vi "Cube_Intensity_png.vi"(3 "No of Contours":i32=20, 4 "Job Directory":path=path "/Lacie_20/paulhayden/Documents/EnFlo bits/EnFlo Tun Vel profiles/View_LDA data.tpt", 5 "Intensity Graph":dbl[][](graph)) -> ()   [LabVIEW 2011]
uses:
  Results_plotter_Global.vi
panel:
  in  "Save Automatically?":bool
  in  "Auto scale Intensity":bool=TRUE
  in  "Colour":bool=TRUE
  out "Results Filename":string
  out "Date":string
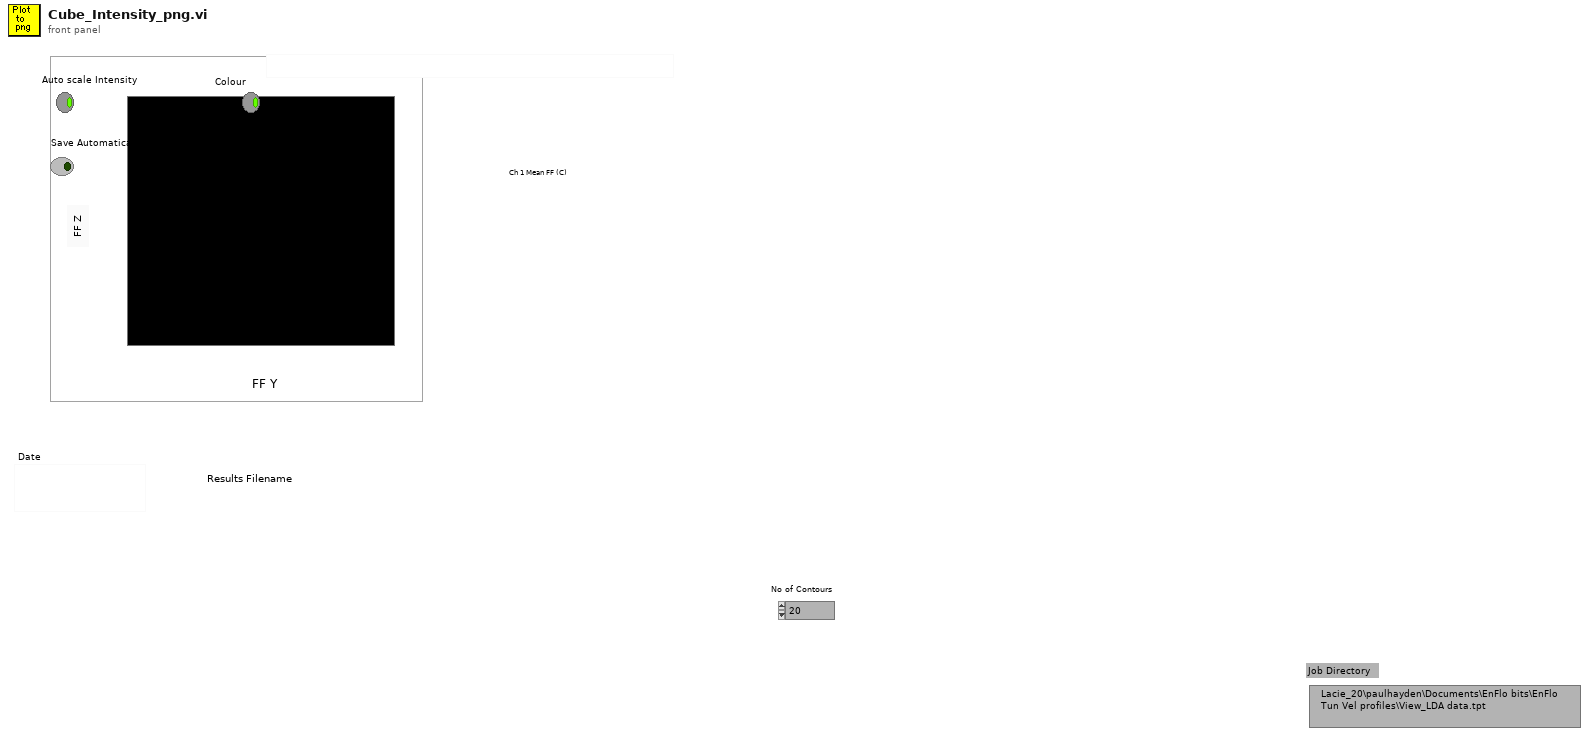
[diagram p1: front panel]
types:
  T1 = typedef "LVRectTypeDef.ctl" = cluster{"left":i16, "top":i16, "right":i16, "bottom":i16}
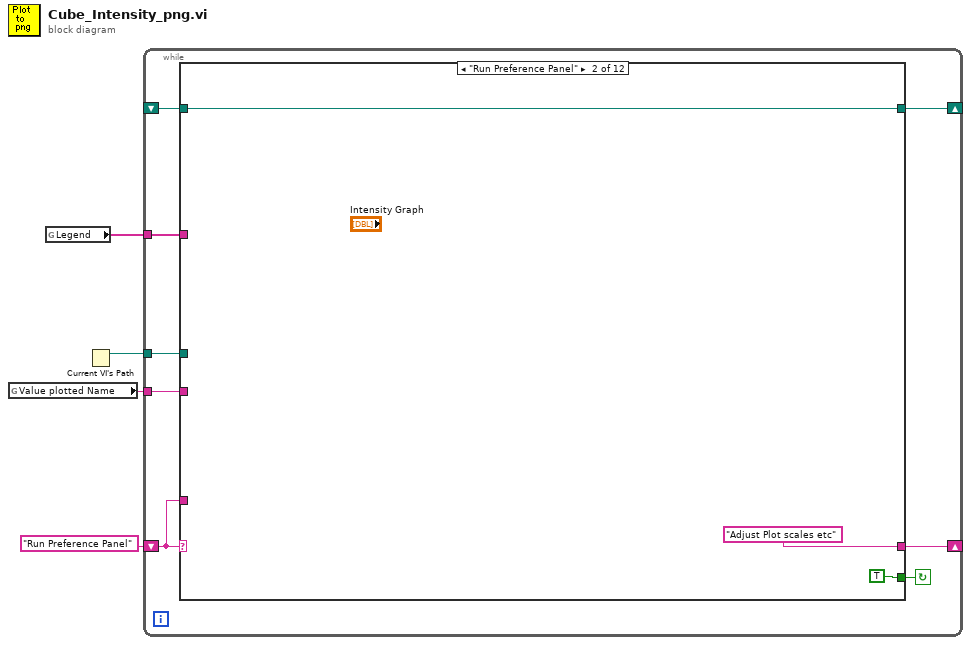
[diagram p0: block diagram]
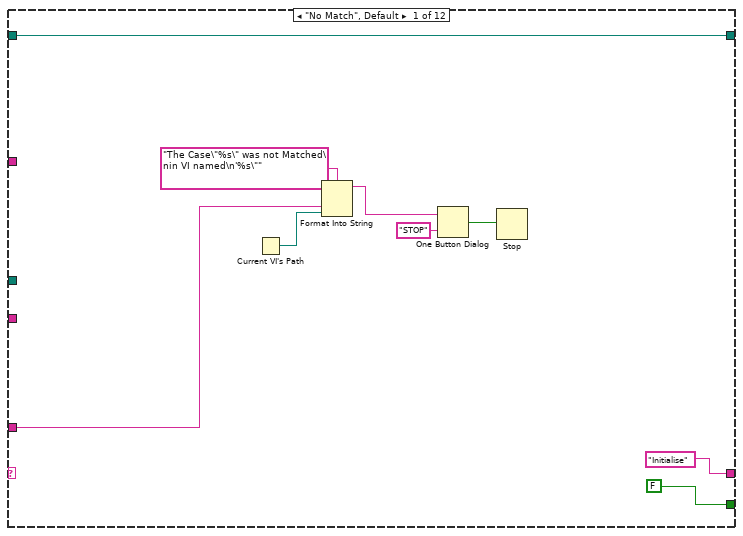
[diagram p2: hidden frame]
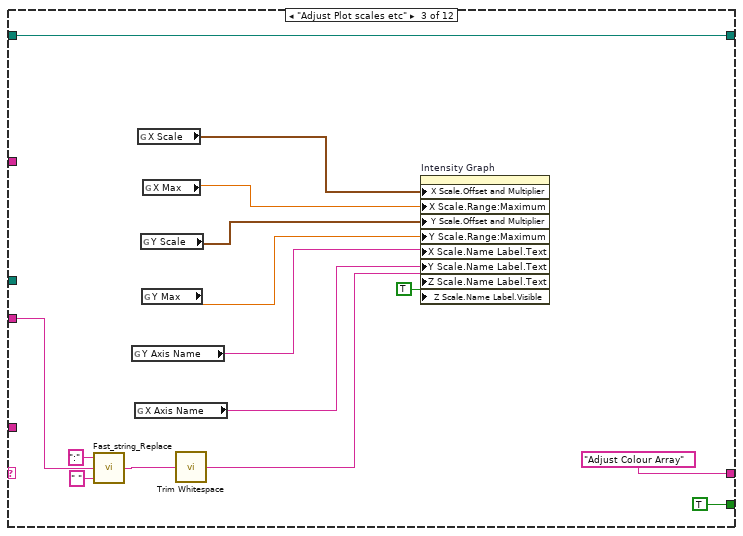
[diagram p3: hidden frame]
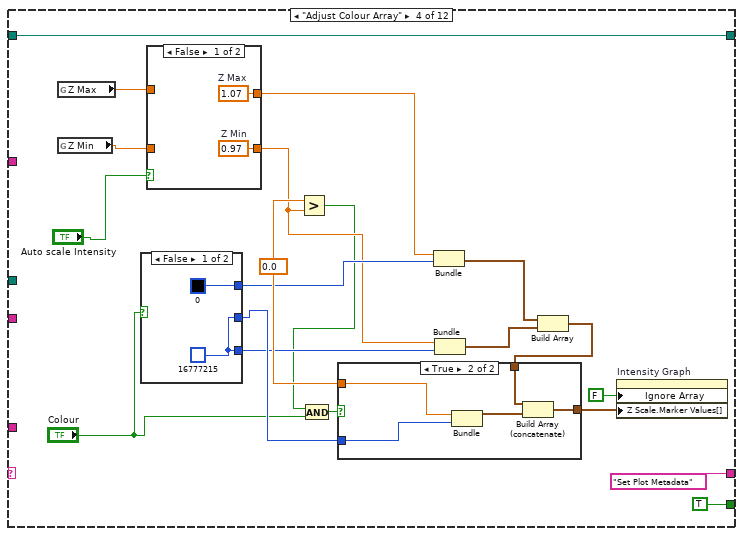
[diagram p4: hidden frame]
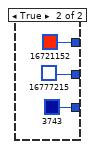
[diagram p5: hidden frame]
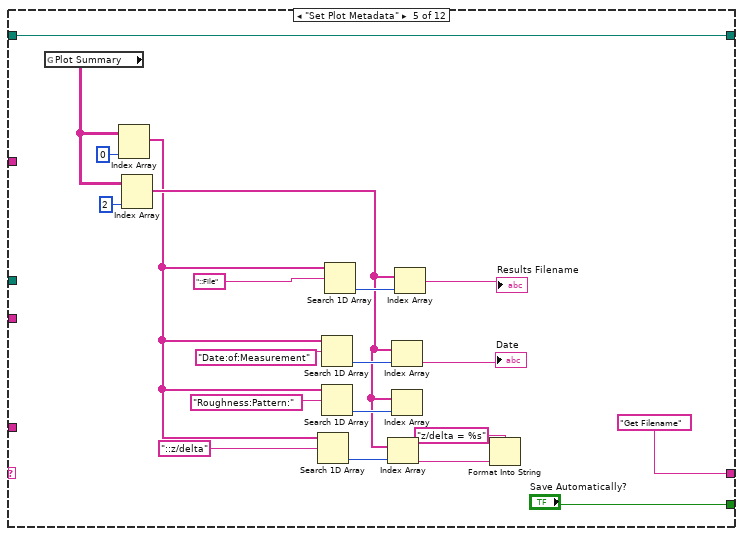
[diagram p8: hidden frame]
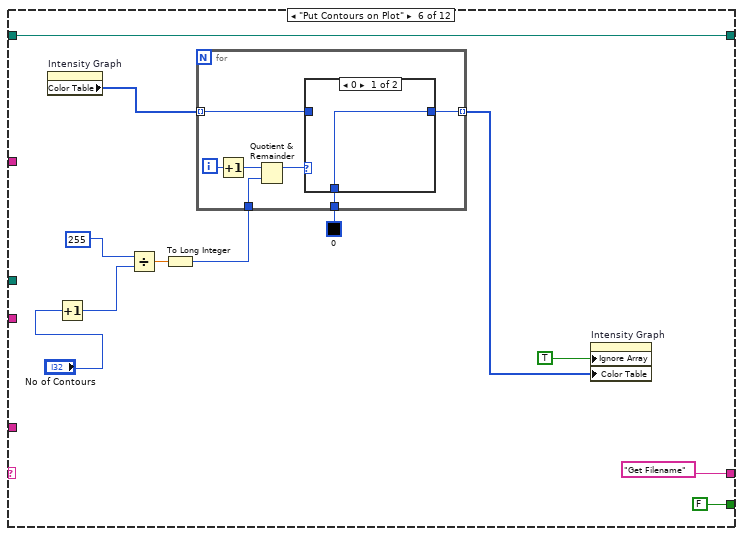
[diagram p9: hidden frame]
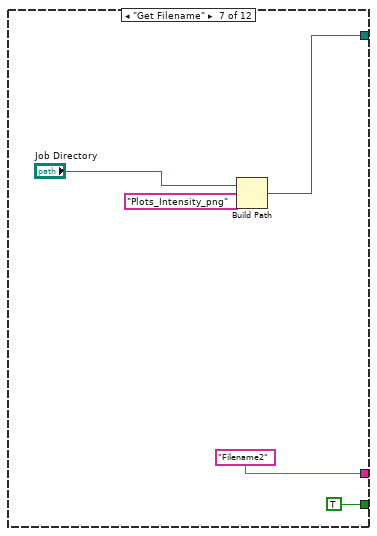
[diagram p11: hidden frame]
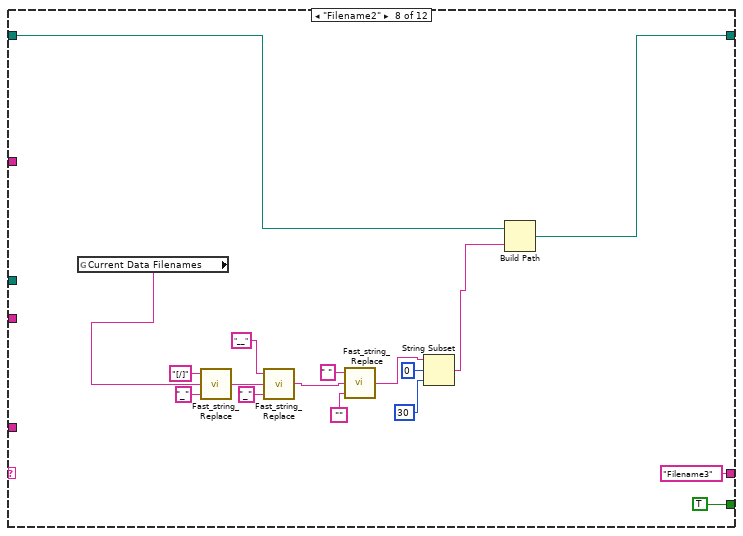
[diagram p12: hidden frame]
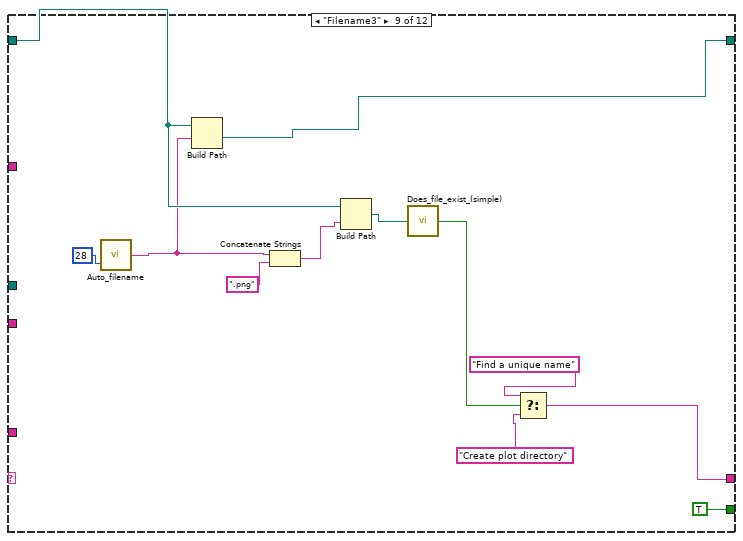
[diagram p13: hidden frame]
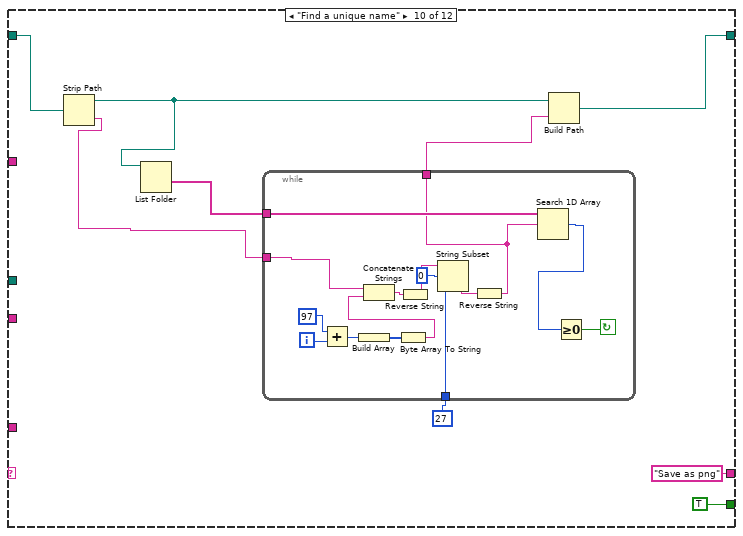
[diagram p14: hidden frame]
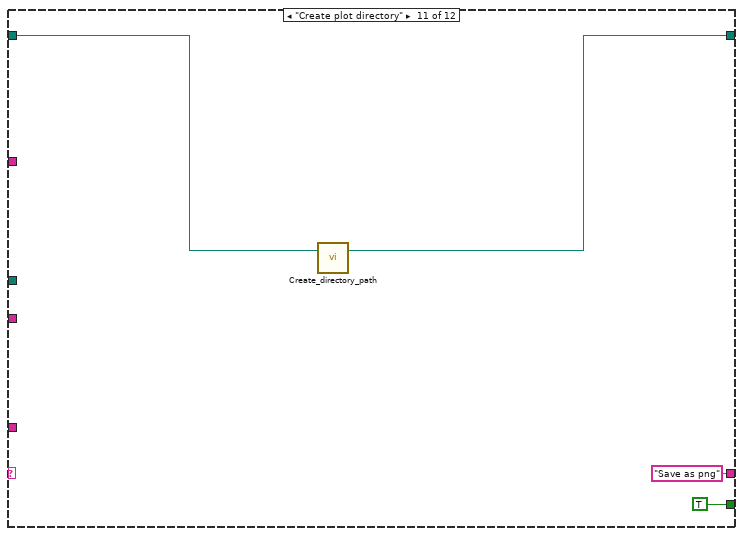
[diagram p15: hidden frame]
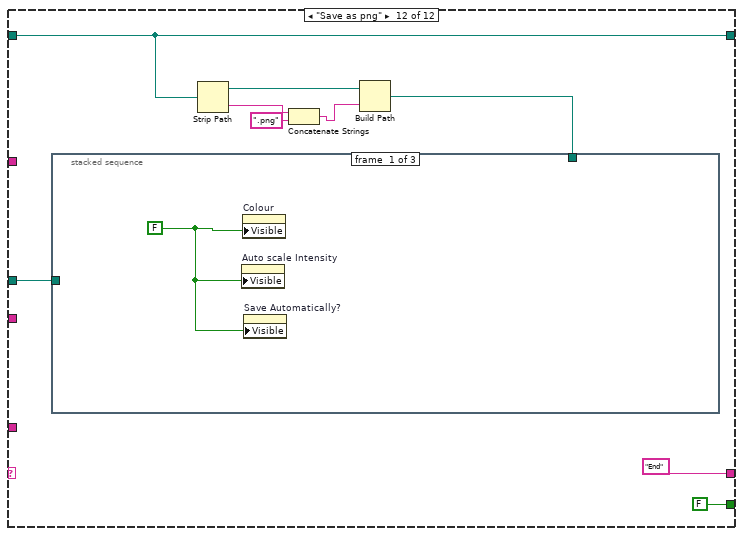
[diagram p16: hidden frame]
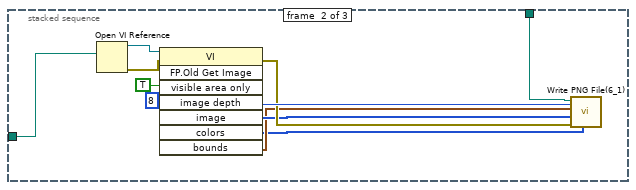
[diagram p17: hidden frame]
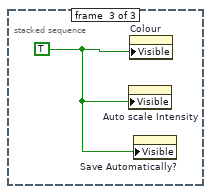
[diagram p18: hidden frame]
diagram:
  n1 = global read "Results_plotter_Global.vi" "Value plotted Name"() -> (w2:string)
  n2 = global read "Results_plotter_Global.vi" "Legend"() -> (w1:string[])
  n3 = Current VI's Path() -> (path=w3:path)
  n4 = while {
    shift-left: "Run Preference Panel" -> [w10]
    shift-right: [w11] -> _
    tunnel: w3 -> [w9]
    shift-right: [w8] -> _
    shift-left: _ -> [w7]
    tunnel: w2 -> [w6]
    tunnel: w1 -> [w5]
    stop <- w12 continue-if-true
    n5 = case shown="\"Run Preference Panel\"" w10 {
      tunnel: [FALSE TRUE TRUE ("Top Level") TRUE ("Top Level") "Save Automatically?" FALSE ("Top Level") TRUE ("Top Level") TRUE ("Top Level") TRUE ("Top Level") TRUE ("Top Level") TRUE ("Top Level") FALSE ("Top Level")] -> w12
      tunnel: ["Initialise" "Adjust Plot scales etc" "Adjust Colour Array" "Set Plot Metadata" "Get Filename" "Get Filename" "Filename2" "Filename3" w146 "Save as png" "Save as png" "End"] -> w11
      tunnel: w10 -> [w16 _ _ _ _ _ _ _ _ _ _ _]
      tunnel: w9 -> [_ _ _ _ _ _ _ _ _ _ _ w185]
      tunnel: [w13 w22 w30 w48 w76 w95 w118 w123 w147 w151 w174 w182] -> w8
      tunnel: w7 -> [w13 w22 w30 w48 w76 w95 _ w124 w148 w152 w175 w182]
      tunnel: w6 -> [_ _ w29 _ _ _ _ _ _ _ _ _]
      tunnel: w5 -> [_ _ _ _ _ _ _ _ _ _ _ _]
      frame "No Match", Default {
        n6 = Current VI's Path() -> (path=w15:path)
        n7 = Format Into String(format string="The Case\"%s\" was not Matched\nin VI named\n'%s\"" ("Format String"), w16, w15) -> (resulting string=w19:string)  [unwired: 2 in, 1 out]
        n8 = One Button Dialog(message=w19, button name ("OK")="STOP") -> (true=w17:bool)
        n9 = Stop(stop? (T)=w17) -> ()
      }
      frame "Run Preference Panel" {
      }
      frame "Adjust Plot scales etc" {
        n10 = call "Fast_string_Replace.vi"("Replace match with:"=" ", "Input String"=w29, "regular expression"=":") -> ("Output String"=w26:string)  [unwired: 1 in, 1 out]
        n11 = global read "Results_plotter_Global.vi" "Y Axis Name"() -> (w33:string)
        n12 = global read "Results_plotter_Global.vi" "X Axis Name"() -> (w32:string)
        n13 = global read "Results_plotter_Global.vi" "X Scale"() -> (w38:cluster{"Xo":dbl, "delta X":dbl})
        n14 = global read "Results_plotter_Global.vi" "Y Scale"() -> (w36:cluster{"Xo":dbl, "delta X":dbl})
        n15 = global read "Results_plotter_Global.vi" "Y Max"() -> (w35:dbl)
        n16 = global read "Results_plotter_Global.vi" "X Max"() -> (w37:dbl)
        n17 = call <vilib>:"Trim Whitespace.vi"("string"=w26) -> ("trimmed string"=w25:string)  [unwired: 1 in]
        n18 = property on="Intensity Graph" class="IntGraph (strict)"("X Scale.Offset and Multiplier"=w38, "X Scale.Range:Maximum"=w37, "Y Scale.Offset and Multiplier"=w36, "Y Scale.Range:Maximum"=w35, "X Scale.Name Label.Text"=w33, "Y Scale.Name Label.Text"=w32, "Z Scale.Name Label.Text"=w25, "Z Scale.Name Label.Visible"=TRUE) -> ()  [unwired: 2 in, 2 out]
      }
      frame "Adjust Colour Array" {
        w59 = 0.0 ("max Z value")
        n19 = global read "Results_plotter_Global.vi" "Z Max"() -> (w46:dbl)
        n20 = global read "Results_plotter_Global.vi" "Z Min"() -> (w44:dbl)
        n21 = case shown="False" "Colour" {
          tunnel: [w61 u32 16777215] -> w55
          tunnel: [u32 0 u32 16721152] -> w54
          tunnel: [w61 u32 3743] -> w50
          frame False {
            w61 = u32 16777215
          }
          frame True {
          }
        }
        n22 = case shown="False" "Auto scale Intensity" {
          tunnel: [w66 w68] -> w47
          tunnel: w46 -> [_ w68]
          tunnel: [w65 w67] -> w45
          tunnel: w44 -> [_ w67]
          frame False {
            w65 = 0.97  # Z Min
            w66 = 1.07  # Z Max
          }
          frame True {
          }
        }
        n23 = Greater?(x=w59, y=w45) -> (0:w42:bool)
        n24 = And(x=w42, y="Colour") -> (x .and. y?=w41:bool)
        n25 = Bundle("Z Max"=w47, w54) -> (w56:cluster{"Z Max":dbl, u32})  [unwired: 1 in]
        n26 = Bundle("Z Min"=w45, w50) -> (w58:cluster{"Z Min":dbl, u32})  [unwired: 1 in]
        n27 = Build Array(w56, w58) -> (w57:cluster{"Z Min":dbl, u32}[])
        n28 = case shown="True" w41 {
          tunnel: w57 -> [w69 w74]
          tunnel: [w69 w72] -> w52
          tunnel: w55 -> [_ w71]
          tunnel: w59 -> [_ w70]
          frame False {
          }
          frame True {
            n29 = Bundle("max Z value"=w70, w71) -> (w73:cluster{"max Z value":dbl, u32})  [unwired: 1 in]
            n30 = Build Array (concatenate)(w74, w73) -> (w72:cluster{"max Z value":dbl, u32}[])
          }
        }
        n31 = property on="Intensity Graph" class="IntGraph (strict)"("Ignore Array"=FALSE, "Z Scale.Marker Values[]"=w52) -> ()  [unwired: 2 in, 2 out]
      }
      frame "Set Plot Metadata" {
        n32 = global read "Results_plotter_Global.vi" "Plot Summary"() -> (w91:string[][])
        n33 = Index Array(array=w91, index (col)=0 ("disabled index (col)")) -> (element=w81:string[])  [unwired: 1 in]
        n34 = Index Array(array=w91, index (col)=2 ("disabled index (col)")) -> (element=w82:string[])  [unwired: 1 in]
        n35 = Search 1D Array(1D array=w81, element="::z/delta") -> (index of element=w85:i32)  [unwired: 1 in]
        n36 = Search 1D Array(1D array=w81, element="Date:of:Measurement") -> (index of element=w87:i32)  [unwired: 1 in]
        n37 = Search 1D Array(1D array=w81, element="Roughness:Pattern:") -> (index of element=w86:i32)  [unwired: 1 in]
        n38 = Search 1D Array(1D array=w81, element="::File") -> (index of element=w90:i32)  [unwired: 1 in]
        n39 = Index Array(array=w82, index=w85) -> (element=w79:string)
        n40 = Index Array(array=w82, index=w87) -> (element=→"Date":string)
        n41 = Index Array(array=w82, index=w86) -> ()  [unwired: 1 out]
        n42 = Index Array(array=w82, index=w90) -> (element=→"Results Filename":string)
        n43 = Format Into String(format string="z/delta = %s", w79) -> ()  [unwired: 2 in, 2 out]
      }
      frame "Put Contours on Plot" {
        n44 = property on="Intensity Graph" class="IntGraph (strict)"() -> ("Color Table"=w98:u32[])  [unwired: 2 in, 2 out]
        n45 = Increment(x="No of Contours") -> (x+1=w103:i32)
        n46 = Divide(x=255, y=w103) -> (x/y=w102:dbl)
        n47 = To Long Integer(number=w102) -> (32bit integer=w100:i32)
        n48 = for {
          tunnel: w100 -> [w112]
          tunnel: [w109] -> w97 mode=indexing
          tunnel: w98 -> [w108] mode=indexing
          tunnel: u32 0 -> [w107]
          i -> [w113]
          n49 = Increment(x=w113) -> (x+1=w110:i32)
          n50 = Quotient & Remainder(x=w110, y=w112) -> (x-y*floor(x/y)=w111:i32)  [unwired: 1 out]
          n51 = case shown="0" w111 {
            tunnel: [w114 w115] -> w109
            tunnel: w108 -> [_ w115]
            tunnel: w107 -> [w114 _]
            frame 0 {
            }
            frame 1, Default {
            }
          }
        }
        n52 = property on="Intensity Graph" class="IntGraph (strict)"("Ignore Array"=TRUE, "Color Table"=w97) -> ()  [unwired: 2 in, 2 out]
      }
      frame "Get Filename" {
        n53 = Build Path(base path="Job Directory", name or relative path="Plots_Intensity_png") -> (appended path=w118:path)
      }
      frame "Filename2" {
        n54 = global read "Results_plotter_Global.vi" "Current Data Filenames"() -> (w135:string)
        n55 = call "Fast_string_Replace.vi"("Replace match with:"="_", "Input String"=w135, "regular expression"="[/]") -> ("Output String"=w131:string)  [unwired: 1 in, 1 out]
        n56 = call "Fast_string_Replace.vi"("Replace match with:"="_", "Input String"=w131, "regular expression"="__") -> ("Output String"=w134:string)  [unwired: 1 in, 1 out]
        n57 = call "Fast_string_Replace.vi"("Replace match with:"="", "Input String"=w134, "regular expression"=" ") -> ("Output String"=w136:string)  [unwired: 1 in, 1 out]
        n58 = String Subset(string=w136, offset (0)=0, length (rest)=30 ("length (rest)")) -> (substring=w137:string)
        n59 = Build Path(base path=w124, name or relative path=w137) -> (appended path=w123:path)
      }
      frame "Filename3" {
        n60 = call "Auto_filename.vi"("Filename Max length"=28) -> ("Filename"=w139:string)  [unwired: 1 in]
        n61 = Build Path(base path=w148, name or relative path=w139) -> (appended path=w147:path)
        n62 = Concatenate Strings(w139, ".png" ("string")) -> (w144:string)
        n63 = Build Path(base path=w148, name or relative path=w144) -> (appended path=w143:path)
        n64 = call "Does_file_exist_(simple).vi"("Pathname"=w143) -> ("exists?"=w142:bool)
        n65 = Select(t="Find a unique name", s=w142, f="Create plot directory") -> (s? t:f=w146:string)
      }
      frame "Find a unique name" {
        n66 = Strip Path(path=w152) -> (stripped path=w150:path, name=w154:string)
        n67 = List Folder(path=w150) -> (folder names=w155:string[])  [unwired: 3 in, 3 out]
        n68 = while {
          tunnel: w154 -> [w173]
          tunnel: 27 ("Max Length") -> [w172]
          tunnel: [w161] -> w156
          tunnel: w155 -> [w162]
          i -> [w163]
          stop <- w159 continue-if-true
          n69 = Add(x=97, y=w163) -> (x+y=w170:i32)
          n70 = Build Array(w170) -> (w171:i32[])
          n71 = Byte Array To String(unsigned byte array=w171) -> (string=w168:string)
          n72 = Concatenate Strings(w173, w168) -> (w166:string)
          n73 = Reverse String(1:w166) -> (0:w167:string)
          n74 = String Subset(string=w167, offset (0)=0, length (rest)=w172) -> (substring=w165:string)
          n75 = Reverse String(1:w165) -> (0:w161:string)
          n76 = Search 1D Array(1D array=w162, element=w161) -> (index of element=w160:i32)  [unwired: 1 in]
          n77 = Greater Or Equal To 0?(x=w160) -> (x >= 0?=w159:bool)
        }
        n78 = Build Path(base path=w150, name or relative path=w156) -> (appended path=w151:path)
      }
      frame "Create plot directory" {
        n79 = call "Create_directory_path.vi"("Path name"=w175) -> ("Path name Out"=w174:path)  [unwired: 1 in, 1 out]
      }
      frame "Save as png" {
        n80 = Strip Path(path=w182) -> (stripped path=w183:path, name=w181:string)
        n81 = Concatenate Strings(w181, ".png" ("string")) -> (w180:string)
        n82 = Build Path(base path=w183, name or relative path=w180) -> (appended path=w178:path)
        n83 = stacked-sequence {
          tunnel: w185 -> [_ w195 _]
          tunnel: w178 -> [_ w188 _]
          frame #0 {
            w187 = FALSE ("Visible")
            n84 = property on="Auto scale Intensity" class="Bool (strict)"("Visible"=w187) -> ()  [unwired: 2 in, 2 out]
            n85 = property on="Colour" class="Bool (strict)"("Visible"=w187) -> ()  [unwired: 2 in, 2 out]
            n86 = property on="Save Automatically?" class="Bool (strict)"("Visible"=w187) -> ()  [unwired: 2 in, 2 out]
          }
          frame #1 {
            w193 = 8 ("image depth")
            n87 = Open VI Reference(vi path=w195) -> (vi reference=w197:refnum<vi>, error out=w196:errorcluster)  [unwired: 5 in]
            n88 = invoke class="VI" method="FP.Old Get Image"(reference=w197, error in=w196, "visible area only"=TRUE, "image depth"=w193) -> (error out=w192:errorcluster, "image"=w191:u8[], "colors"=w189:u32[], "bounds"=w190:T1)  [unwired: 4 in, 4 out]
            n89 = call <vilib>:"Write PNG File(6_1).vi"("color table"=w189, "depth"=w193, "error in (no error)"=w192, "flattened image data"=w191, "rect"=w190, "path to PNG file"=w188) -> ()  [unwired: 4 in, 2 out]
          }
          frame #2 {
            w198 = TRUE ("Visible")
            n90 = property on="Auto scale Intensity" class="Bool (strict)"("Visible"=w198) -> ()  [unwired: 2 in, 2 out]
            n91 = property on="Colour" class="Bool (strict)"("Visible"=w198) -> ()  [unwired: 2 in, 2 out]
            n92 = property on="Save Automatically?" class="Bool (strict)"("Visible"=w198) -> ()  [unwired: 2 in, 2 out]
          }
        }
      }
    }
  }
